vi "ballBBack.vi"(10 "클러스터":T1, 11 "ColorSensor":dbl[](array[numeric])) -> ()   [LabVIEW 2014]
panel:
  in  "왼쪽으로 빠지는 초":u32=800
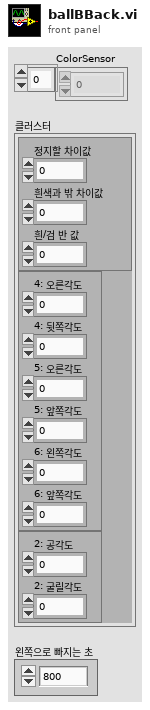
[diagram p1: front panel]
types:
  T1 = cluster{cluster{"정지할 차이값":dbl, "흰색과 밖 차이값":dbl, "흰/검 반 값 ":dbl}, cluster{"4: 오른각도":dbl, "4: 뒷쪽각도":dbl, "5: 오른각도":dbl, "5: 앞쪽각도":dbl, "6: 왼쪽각도":dbl, "6: 앞쪽각도":dbl}, cluster{"2: 공각도":dbl, "2: 굴릴각도":dbl}}
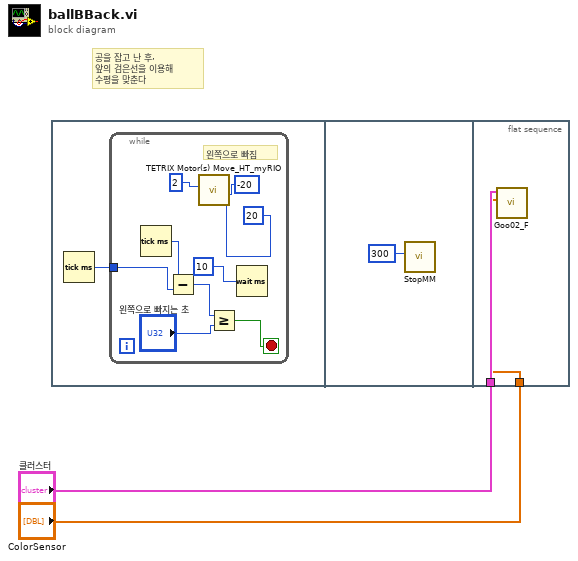
[diagram p0: block diagram]
diagram:
  # "공을 잡고 난 후,\n앞의 검은선을 이용해\n수평을 맞춘다"
  n1 = flat-sequence {
    tunnel: "클러스터" -> [w15]
    tunnel: "ColorSensor" -> [w14]
    frame #0 {
      n2 = Tick Count (ms)() -> (millisecond timer value=w3:u32)
      n3 = while {
        tunnel: w3 -> [w8]
        stop <- w7 stop-if-true
        # "왼쪽으로 빠짐"
        n4 = Tick Count (ms)() -> (millisecond timer value=w9:u32)
        n5 = Subtract(x=w9, y=w8) -> (x-y=w6:u32)
        n6 = call <vilib>:"TETRIX Motor(s) Move_HT_myRIO.vi"("Motor 2 Power (-100 to 100)\n0 = Stop/Brake\n-128 = Stop/Coast"=i8 20 ("Motor 2 Power (-100 to 100)\n0 = Stop/Brake\n-128 = Stop/Coast"), "Motor 1 Power (-100 to 100)\n0 = Stop/Brake\n-128 = Stop/Coast"=i8 -20 ("Motor 1 Power (-100 to 100)\n0 = Stop/Brake\n-128 = Stop/Coast"), "Controller Daisy Chain Position: 1 - 4"=u8 2) -> ()  [unwired: 6 in, 1 out]
        n7 = Greater Or Equal?(x=w6, y="왼쪽으로 빠지는 초") -> (x >= y?=w7:bool)
        n8 = Wait (ms)(milliseconds to wait=u32 10 ("대기 시간(ms)")) -> ()  [unwired: 1 out]
      }
    }
    frame #1 {
      n9 = call "StopMM.vi"("대기 시간(ms)"=u32 300) -> ()  [unwired: 11 in]
    }
    frame #2 {
      n10 = call "Goo02_F.vi"("ColorSensor 2"=w14, "클러스터"=w15) -> ()  [unwired: 10 in]
    }
  }
